vi "管理机电流判断.vi"(1 "数值":dbl format="%.1g") -> (0 "s? t:f":dbl)   [LabVIEW 2015]
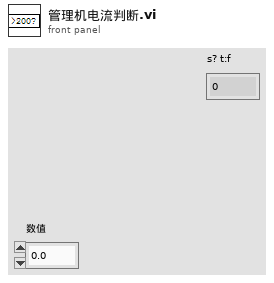
[diagram p1: front panel]
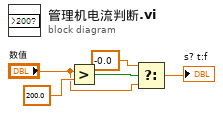
[diagram p0: block diagram]
diagram:
  n1 = Greater?(x="数值", y=200.0) -> (0:w4:bool)
  n2 = Select(t=-0.0, s=w4, f="数值") -> (s? t:f=→"s? t:f":dbl)
